vi "Set Dispenser State.vi"(8 "error in":errorcluster, 10 "On/Off":bool, 11 "Gantry in":refnum<class "Gantry.lvclass">) -> (0 "error out":errorcluster, 3 "Gantry out":refnum<class "Gantry.lvclass">)   [LabVIEW 2017, in "Gantry.lvclass"]
uses:
  Gantry.lvclass
  Gantry.lvclass/Gantry.ctl
  <vilib>/DAQmx/write.llb/DAQmx Write (Digital Bool 1Line 1Point).vi
  <vilib>/DAQmx/miscellaneous.llb/DAQmx Fill In Error Info.vi
  FlexWorktable/FlexWorktable.lvclass
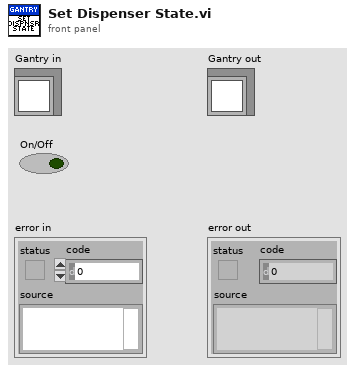
[diagram p1: front panel]
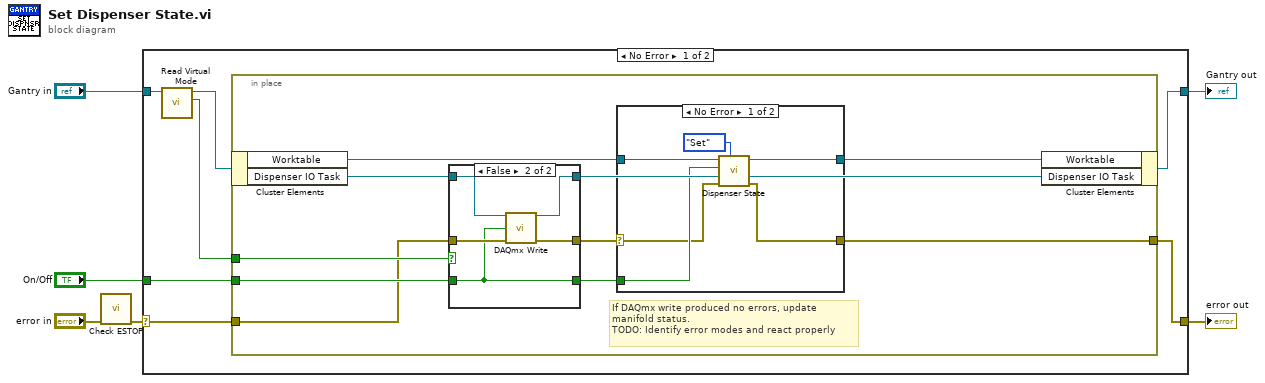
[diagram p0: block diagram]
diagram:
  n1 = call "Check ESTOP.vi"("error in"="error in") -> ("error out"=w2:errorcluster)  [unwired: 10 in]
  n2 = case shown="No Error" w2 {
    selector: w2 -> [w12 w41]
    tunnel: [w10 w41] -> w6
    tunnel: [w11 w40] -> w5
    tunnel: "Gantry in" -> [w9 w40]
    tunnel: "On/Off" -> [w13 _]
    frame No Error {
      n3 = call-dynamic "Read Virtual Mode.vi"("Gantry in"=w9) -> ("Is Virtual"=w7:bool, "Gantry out"=w8:refnum<class "Gantry.lvclass">)  [unwired: 7 in, 2 out]
      n4 = in-place {
        in-place-border: w13 -> [w20]
        in-place-border: w12 -> [w17]
        in-place-border: [w14] -> w10
        in-place-border: w7 -> [w18]
        # "If DAQmx write produced no errors, update \nmanifold status.\nTODO: Identify error modes and react properly"
        n5 = in-place-cluster #1(w8) -> ("Worktable"=w16:refnum<class "FlexWorktable.lvclass">, "Dispenser IO Task"=w22:refnum<k21>)
        n6 = case shown="False" w18 {
          tunnel: [w25 w31] -> w23
          tunnel: w22 -> [w26 w30]
          tunnel: [w26 w29] -> w21
          tunnel: w20 -> [w24 w27]
          tunnel: w17 -> [w25 w28]
          tunnel: [w24 w27] -> w19
          frame True {
          }
          frame False {
            n7 = call-poly <vilib>:"DAQmx Write.vi"("task/channels in"=w30, "data"=w27, "error in"=w28) -> ("task out"=w29:refnum<k21>, "error out"=w31:errorcluster)  [unwired: 10 in, 1 out]
          }
        }
        n8 = case shown="No Error" w23 {
          selector: w23 -> [w34 w39]
          tunnel: w19 -> [w37 _]
          tunnel: [w32 w39] -> w14
          tunnel: w16 -> [w36 w38]
          tunnel: [w35 w38] -> w15
          frame No Error {
            n9 = call-dynamic "Dispenser State.vi"("Get/Set"=enum16{"Get", "Set"}."Set", "error in (no error)"=w34, "New State"=w37, "FlexWorktable in"=w36) -> ("error out"=w32:errorcluster, "FlexWorktable out"=w35:refnum<class "FlexWorktable.lvclass">)  [unwired: 5 in, 1 out]
          }
          frame Error {
          }
        }
        n10 = in-place-cluster #1("Worktable"=w15, "Dispenser IO Task"=w21) -> (w11:refnum<class "Gantry.lvclass">)
      }
    }
    frame Error {
    }
  }
  "error out" <- w6
  "Gantry out" <- w5
